vi "Create Assert VI.vi"(6 "Assert VI path":path, 7 "Type":T1, 8 "error in (no error)":errorcluster, 10 "Template Path":path) -> (0 "error out":errorcluster)   [LabVIEW 2018]
doc: "Creates a new vi based on the specified template and saves it to the new path"
uses:
  <vilib>/Utility/Data Type/Type Definitions/Data Type.ctl
  <vilib>/Utility/Data Type/NI_Data Type.lvlib
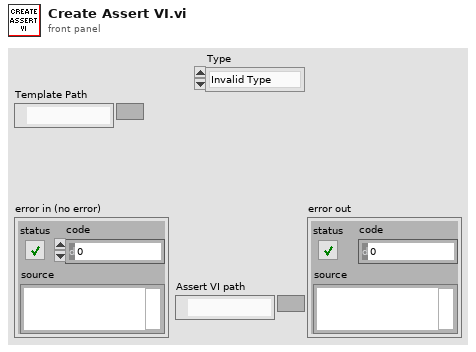
[diagram p1: front panel]
types:
  T1 = typedef "NI_Data Type.lvlib/Data Type.ctl" = enum8{"Invalid Type", "Void", "I8", "I16", "I32", "I64", "U8", "U16", "U32", "U64", "Single Float", "Double Float", "Extended Float", "Single Complex", "Double Complex", "Extended Complex", "Enum U8", "Enum U16", "Enum U32", "Enum U64", "Single Float With Unit", "Double Float With Unit", "Extended Float With Unit", "Single Complex with Unit", "Double Complex with Unit", "Extended Complex with Unit", "Boolean", "String", "Path", "Picture", "Tag", "Array", "Cluster", "Variant", "LV Variant", "Waveform", "Timestamp", "Digital Waveform", "Digital Data", "ExpressData", "Refnum", "External Data", "VI", "Poly VI", "LabVIEW Class Instance", "Fixed Point"}
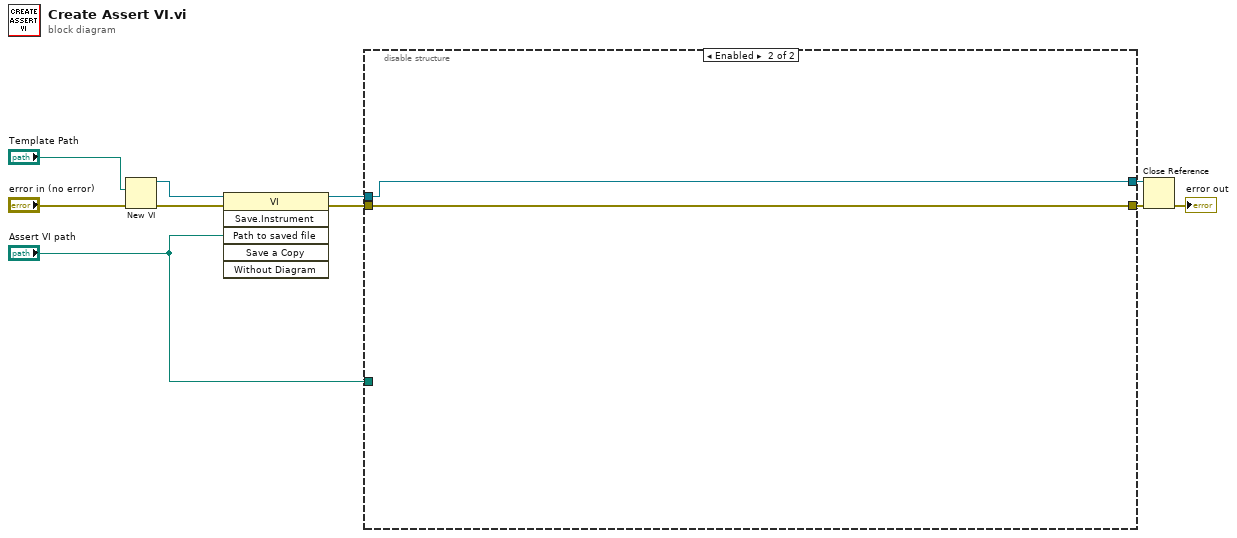
[diagram p0: block diagram]
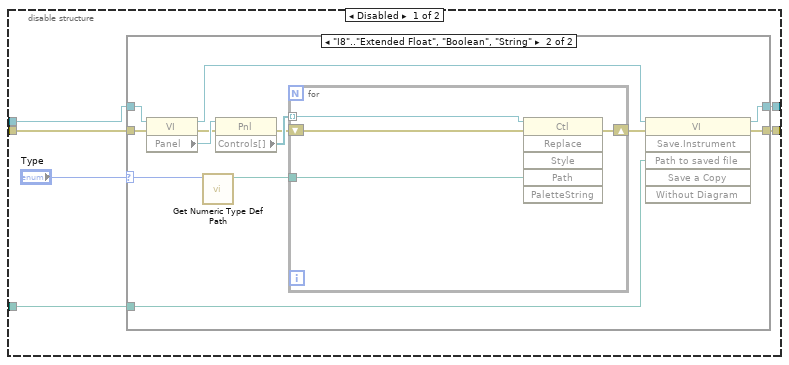
[diagram p2: hidden frame]
diagram:
  n1 = New VI(8:"error in (no error)", 10:"Template Path") -> (0:w7:errorcluster, 3:w6:refnum<vi>)  [unwired: 5 in]
  n2 = invoke class="VI" method="Save.Instrument"(reference=w6, error in=w7, "Path to saved file"="Assert VI path") -> (reference out=w4:refnum<vi>, error out=w2:errorcluster)  [unwired: 3 in, 4 out]
  n3 = disable-structure shown="Enabled" {
    disable-tunnel: [w16 w37] -> w5
    disable-tunnel: w4 -> [w15 w37]
    disable-tunnel: [w14 w36] -> w3
    disable-tunnel: w2 -> [w13 w36]
    disable-tunnel: "Assert VI path" -> [w12 _]
    frame Disabled {
      n4 = case shown="\"I8\"..\"Extended Float\", \"Boolean\", \"String\"" "Type" {
        selector: "Type" -> [_ w20]
        tunnel: [w18 w22] -> w16
        tunnel: w15 -> [w18 w31]
        tunnel: [w17 w24] -> w14
        tunnel: w13 -> [w17 w25]
        tunnel: w12 -> [_ w21]
        frame Default {
        }
        frame "I8".."Extended Float", "Boolean", "String" {
          n5 = property class="VI"(reference=w31, error in=w25) -> (reference out=w23:refnum<vi>, error out=w26:errorcluster, "Panel"=w30:refnum<vi>)
          n6 = call "Get Numeric Type Def Path.vi"("Type"=w20) -> ("Numeric Type Def Path"=w19:path)  [unwired: 9 in, 1 out]
          n7 = property class="Pnl"(reference=w30, error in=w26) -> (error out=w27:errorcluster, "Controls[]"=w29:refnum<vi>[])  [unwired: 1 out]
          n8 = for {
            tunnel: w29 -> [w35] mode=indexing
            shift-right: [w34] -> w28
            shift-left: w27 -> [w33]
            tunnel: w19 -> [w32]
            n9 = invoke class="Ctl" method="Replace"(reference=w35, error in=w33, "Path"=w32) -> (error out=w34:errorcluster)  [unwired: 3 in, 5 out]
          }
          n10 = invoke class="VI" method="Save.Instrument"(reference=w23, error in=w28, "Path to saved file"=w21) -> (reference out=w22:refnum<vi>, error out=w24:errorcluster)  [unwired: 3 in, 4 out]
        }
      }
    }
    frame Enabled {
    }
  }
  n11 = Close Reference(reference=w5, error in (no error)=w3) -> (error out=→"error out":errorcluster)
